vi "leebinario_bloque.vi"() -> ()   [LabVIEW 2015]
panel:
  in  "Frecuencia\nmuestreo":dbl=25600.0
  in  "Nº WS":i32=2
  in  "Nº acel":i32=8
  out "T, v, UT":sgl[](array[numeric])
  out "Waveform Graph":waveform(sgl)[](graph)
  in  "Folder Path":path
  out "error out":errorcluster
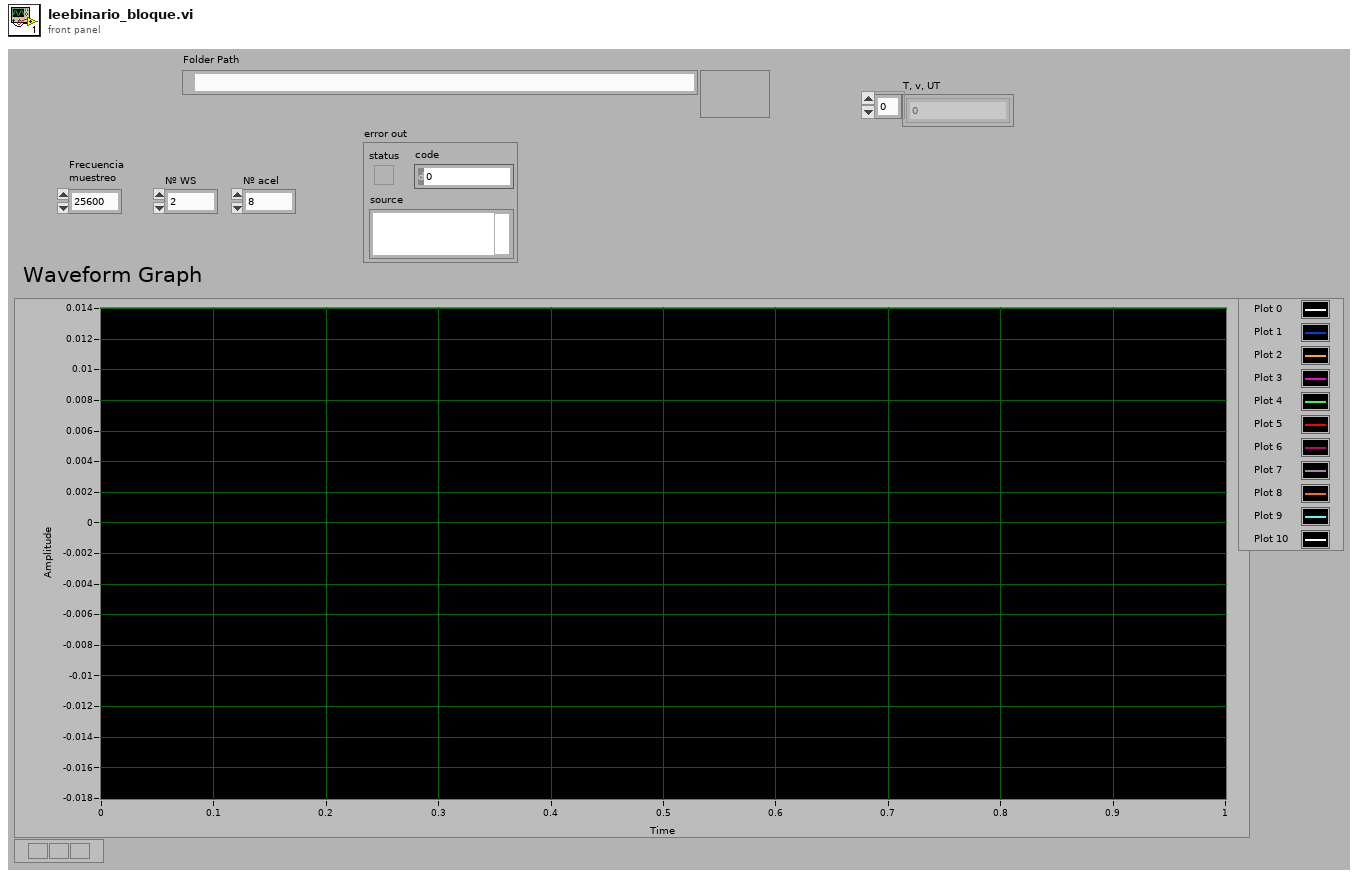
[diagram p1: front panel]
types:
  T1 = enum16{"big-endian, network order", "native, host order", "little-endian"}
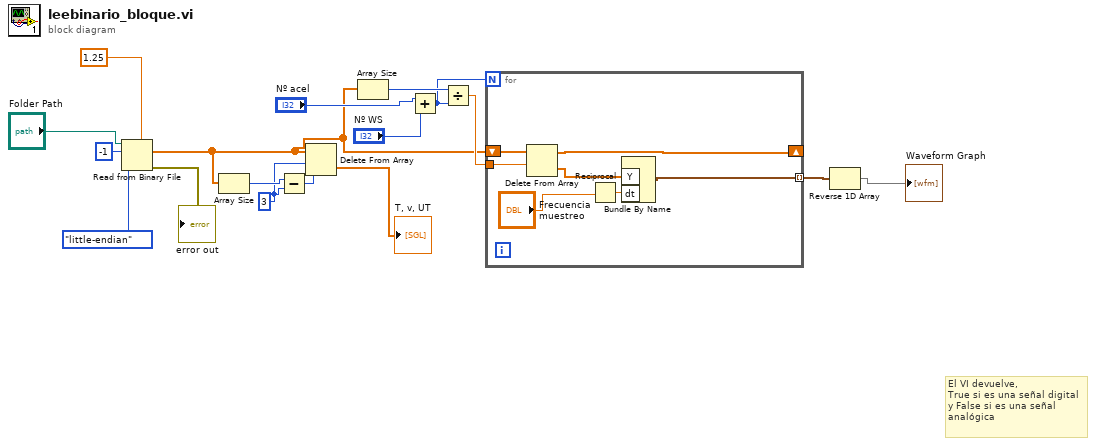
[diagram p0: block diagram]
diagram:
  w11 = 3 ("length")
  # "El VI devuelve,\nTrue si es una señal digital\ny False si es una señal\nanalógica"
  n1 = Read from Binary File(5:sgl 1.25, 9:T1."little-endian" ("byte order (0:big-endian, network order)"), 10:-1 ("count (1)"), 11:"Folder Path") -> (0:→"error out":errorcluster, 2:w2:sgl[])  [unwired: 1 in, 3 out]
  n2 = Array Size(array=w2) -> (size(s)=w13:i32)
  n3 = Subtract(x=w13, y=w11) -> (x-y=w12:i32)
  n4 = Delete From Array(array=w2, length=w11, index=w12) -> (deleted portion=→"T, v, UT":sgl[])  [unwired: 1 out]
  n5 = Array Size(array=w2) -> (size(s)=w10:i32)
  n6 = Add(x="Nº acel", y="Nº WS") -> (x+y=w5:i32)
  n7 = Divide(x=w10, y=w5) -> (x/y=w9:dbl)
  n8 = for {
    N: w5 -> [_]
    tunnel: [w24] -> w1 mode=indexing
    shift-right: [w21] -> _
    shift-left: w2 -> [w22]
    tunnel: w9 -> [w20]
    n9 = Delete From Array(array=w22, length=w20) -> (deleted portion=w18:sgl[], array with subset deleted=w21:sgl[])  [unwired: 1 in]
    n10 = Reciprocal(x="Frecuencia\nmuestreo") -> (1/x=w23:dbl)
    n11 = Bundle By Name("Y"=w18, "dt"=w23) -> (w24:waveform(sgl))  [unwired: 1 in]
  }
  n12 = Reverse 1D Array(array=w1) -> (reversed array=→"Waveform Graph":waveform(sgl)[])
